vi "find_maxes.vi"(0 "Wavelengths":dbl[](array[numeric]), 1 "Trace (r=wl, c=d)":dbl[][](array[numeric]), 2 "Deltas":dbl[](array[numeric]), 3 "Gamma":dbl, 4 "WL central":dbl) -> (5 "Bounds":dbl[][](array[numeric]), 6 "Maxes":dbl[][](array[numeric]))   [LabVIEW 2022 SP3]
panel:
  # "compute delta_m as i*increment"
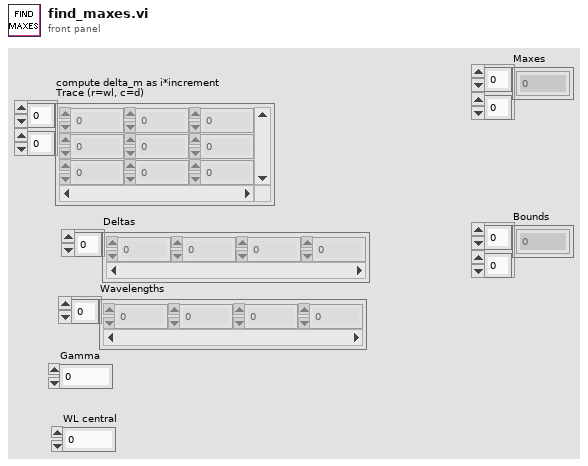
[diagram p1: front panel]
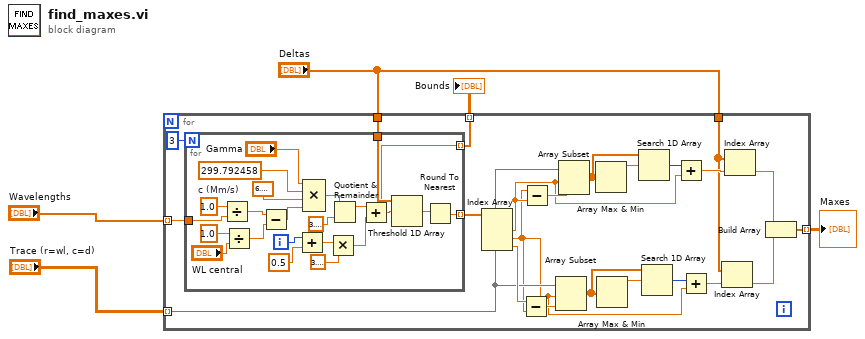
[diagram p0: block diagram]
diagram:
  n1 = for {
    tunnel: "Trace (r=wl, c=d)" -> [w23] mode=indexing
    tunnel: "Wavelengths" -> [w28] mode=indexing
    tunnel: "Deltas" -> [w14]
    tunnel: "Deltas" -> [w11]
    tunnel: [w8] -> w1 mode=indexing
    tunnel: [w6] -> w2 mode=indexing
    n2 = for {
      N: 3 -> [_]
      tunnel: w28 -> [w46]
      tunnel: [w35] -> w7 mode=indexing
      tunnel: w14 -> [w34]
      tunnel: [w29] -> w6 mode=indexing
      i -> [w40]
      w49 = 299.792458  # c (Mm/s)
      n3 = Divide(x=1.0, y=w46) -> (x/y=w44:dbl)
      n4 = Divide(x=1.0, y="WL central") -> (x/y=w41:dbl)
      n5 = Subtract(x=w44, y=w41) -> (x-y=w45:dbl)
      n6 = Add(x=w40, y=0.5) -> (x+y=w38:dbl)
      n7 = Compound Arithmetic op=MULTIPLY("Gamma", w49, 6.283185307179586, w45) -> (w33:dbl)
      n8 = Multiply(x=w38, y=3.141592653589793) -> (x*y=w30:dbl)
      n9 = Quotient & Remainder(x=w33, y=3.141592653589793) -> (x-y*floor(x/y)=w31:dbl)  [unwired: 1 out]
      n10 = Add(x=w31, y=w30) -> (x+y=w29:dbl)
      n11 = Threshold 1D Array(2:w29, 3:w34) -> (0:w36:dbl)  [unwired: 1 in]
      n12 = Round To Nearest(number=w36) -> (nearest integer value=w35:dbl)
    }
    n13 = Index Array(array=w7) -> (element #1=w17:dbl, element #2=w15:dbl, element #3=w25:dbl)  [unwired: 3 in]
    n14 = Subtract(x=w25, y=w15) -> (x-y=w26:dbl)
    n15 = Subtract(x=w15, y=w17) -> (x-y=w24:dbl)
    n16 = Array Subset(array=w23, index=w15, length=w26) -> (w20:dbl[])
    n17 = Array Subset(array=w23, index=w17, length=w24) -> (w22:dbl[])
    n18 = Array Max & Min(array=w22) -> (max value=w21:dbl)  [unwired: 3 out]
    n19 = Array Max & Min(array=w20) -> (max value=w19:dbl)  [unwired: 3 out]
    n20 = Search 1D Array(1D array=w22, element=w21) -> (index of element=w18:i32)  [unwired: 1 in]
    n21 = Search 1D Array(1D array=w20, element=w19) -> (index of element=w16:i32)  [unwired: 1 in]
    n22 = Add(x=w18, y=w17) -> (x+y=w13:dbl)
    n23 = Add(x=w16, y=w15) -> (x+y=w12:dbl)
    n24 = Index Array(array=w11, index=w12) -> (element=w9:dbl)
    n25 = Index Array(array=w11, index=w13) -> (element=w10:dbl)
    n26 = Build Array(w10, w9) -> (w8:dbl[])
  }
  "Bounds" <- w2
  "Maxes" <- w1
